vi "Excel_Insert_Link.vi"(4 "column":i32=1, 5 "name":string, 6 "row":i32=1, 7 "font":T1 {"font size" format="%0.2f"; "strike through" items=["Strk Unchanged", "Strk Yes", "Strk No"]; "underline" items=["Und Unchanged", "Und Yes", "Und No"]; "italic" items=["Ital Unchanged", "Ital Yes", "Ital No"]; "bold" items=["Bold Unchanged", "Bold Yes", "Bold No"]}, 8 "error in (no error)":errorcluster, 9 "text to display":string, 10 "address":string, 11 "worksheet in":refnum<k7>) -> (0 "error out":errorcluster)   [LabVIEW 2017, in "NI_ReportGenerationToolkit.lvlib"]
uses:
  <vilib>/addons/_office/NI_ReportGenerationToolkit.lvlib
  <vilib>/addons/_office/_exclsub.llb/font.ctl
panel:
  in  "Excel.Hyperlink":refnum<k7>
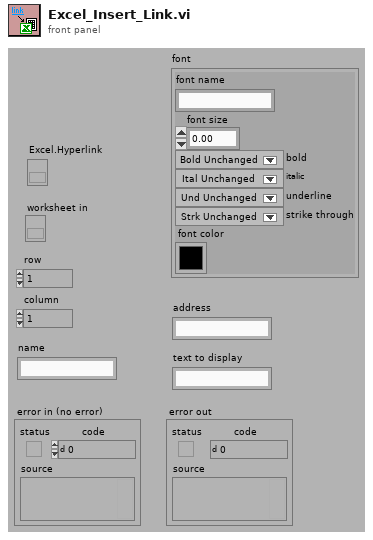
[diagram p1: front panel]
types:
  T1 = typedef "NI_ReportGenerationToolkit.lvlib/font.ctl" = cluster{"font name":string, "font size":dbl, "bold":u16, "italic":u16, "underline":u16, "strike through":u16, "font color":u32}
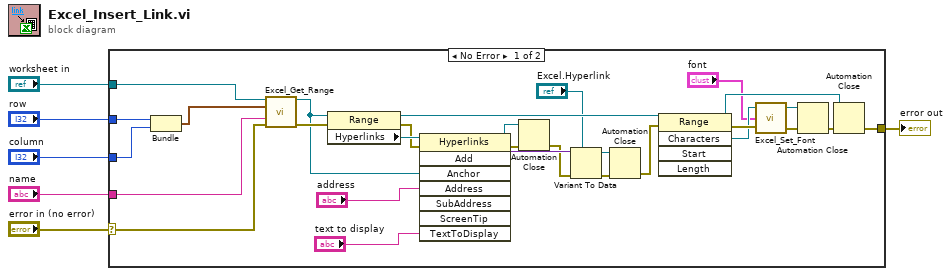
[diagram p0: block diagram]
diagram:
  n1 = case shown="No Error" "error in (no error)" {
    selector: "error in (no error)" -> [w7 w36]
    tunnel: "worksheet in" -> [w29 _]
    tunnel: [w21 w36] -> w5
    tunnel: "name" -> [w11 _]
    tunnel: "column" -> [w10 _]
    tunnel: "row" -> [w9 _]
    frame No Error {
      n2 = Bundle("row"=w9, "column"=w10) -> (w8:cluster{"row":i32, "column":i32})  [unwired: 1 out]
      n3 = call <vilib>:"Excel_Get_Range.vi"("Excel._Worksheet"=w29, "start"=w8, "name"=w11, "error in (no error)"=w7) -> ("Range"=w12:refnum<k7>, "error out"=w35:errorcluster)  [unwired: 1 in, 9 out]
      n4 = property class="Range"(reference=w12, error in=w35) -> (reference out=w27:refnum<k7>, error out=w33:errorcluster, "Hyperlinks"=w34:refnum<k7>)
      n5 = invoke class="Hyperlinks" method="Add"(reference=w34, error in=w33, "Anchor"=w12, "Address"="address", "TextToDisplay"="text to display") -> (reference out=w32:refnum<k7>, error out=w28:errorcluster, "Add"=w18:variant)  [unwired: 3 in, 5 out]
      n6 = Automation Close(3:w28, 5:w32) -> (0:w16:errorcluster)
      n7 = Variant To Data(error in=w16, type="Excel.Hyperlink", Variant=w18) -> (data=w14:refnum<k7>, error out=w15:errorcluster)
      n8 = Automation Close(3:w15, 5:w14) -> (0:w13:errorcluster)
      n9 = invoke class="Range" method="Characters"(reference=w27, error in=w13) -> (reference out=w20:refnum<k7>, error out=w26:errorcluster, "Characters"=w25:refnum<k7>)  [unwired: 3 in, 2 out]
      n10 = call <vilib>:"Excel_Set_Font.vi"("Excel.Characters"=w25, "font"="font", "error in (no error)"=w26) -> ("Excel.Characters out"=w23:refnum<k7>, "error out"=w24:errorcluster)  [unwired: 5 out]
      n11 = Automation Close(3:w24, 5:w23) -> (0:w22:errorcluster)
      n12 = Automation Close(3:w22, 5:w20) -> (0:w21:errorcluster)
    }
    frame Error {
    }
  }
  "error out" <- w5
